vi "选择补传参数对话框.vi"() -> (3 "参数数值 2":T1)   [LabVIEW 2016, in "数据传输系统-02.lvlib"]
uses:
  <vilib>/Utility/miscctls.llb/LVPointTypeDef.ctl
panel:
  in  "取消全选":bool
  in  "取消":bool
  in  "确定":bool
  in  "全选":bool
  in  "参数数值":T2={"CODMn"=TRUE, "CODCr"=TRUE, "DO"=TRUE, "铜"=TRUE, "PH"=TRUE, "氨氮"=TRUE, "比电导率"=TRUE, "水温"=TRUE, "COD"=TRUE, "浊度"=TRUE, "总氮"=TRUE, "总磷"=TRUE, "叶绿素a"=TRUE, "藻密度"=TRUE, "水位"=TRUE, "流速"=TRUE, "瞬时流量"=TRUE, "累积流量"=TRUE, "亚硝氮"=TRUE, "硫化物"=TRUE, "ORP"=TRUE, "铅"=TRUE, "镉"=TRUE, "锌"=TRUE, "镍"=TRUE, "锰"=TRUE, "汞"=TRUE, "气温"=TRUE, "气压"=TRUE, "风速"=TRUE, "风向"=TRUE, "盐度"=TRUE, "磷酸盐"=TRUE, "硝氮"=TRUE, "氟化物"=TRUE, "挥发酚"=TRUE, "氯化物"=TRUE, "蓝绿藻"=TRUE, "余氯"=TRUE, "空气温度"=TRUE, "相对湿度"=TRUE, "分钟雨量"=TRUE, "小时雨量"=TRUE, "日雨量"=TRUE, "累积雨量"=TRUE, "方向"=TRUE, "正累积流量"=TRUE, "负累积流量"=TRUE, "综合生物毒性"=TRUE, "艏向"=TRUE, "横摇"=TRUE, "纵摇"=TRUE, "分层标志"=TRUE, "层状态1"=TRUE, "层状态2"=TRUE, "水平平均流速"=TRUE, "流向"=TRUE, "北向流速分量"=TRUE, "东向流速分量"=TRUE, "垂直流速分量"=TRUE, "最大波高"=TRUE, "最大波周期"=TRUE, "1/10波高"=TRUE, "1/10波周期"=TRUE, "有效波高"=TRUE, "有效波周期"=TRUE, "平均波高"=TRUE, "平均波周期"=TRUE, "波向"=TRUE, "波个数"=TRUE, "水深"=TRUE, "X轴流速"=TRUE, "Y轴流速"=TRUE, "信号强度"=TRUE, "电压"=TRUE, "悬浮物"=TRUE}
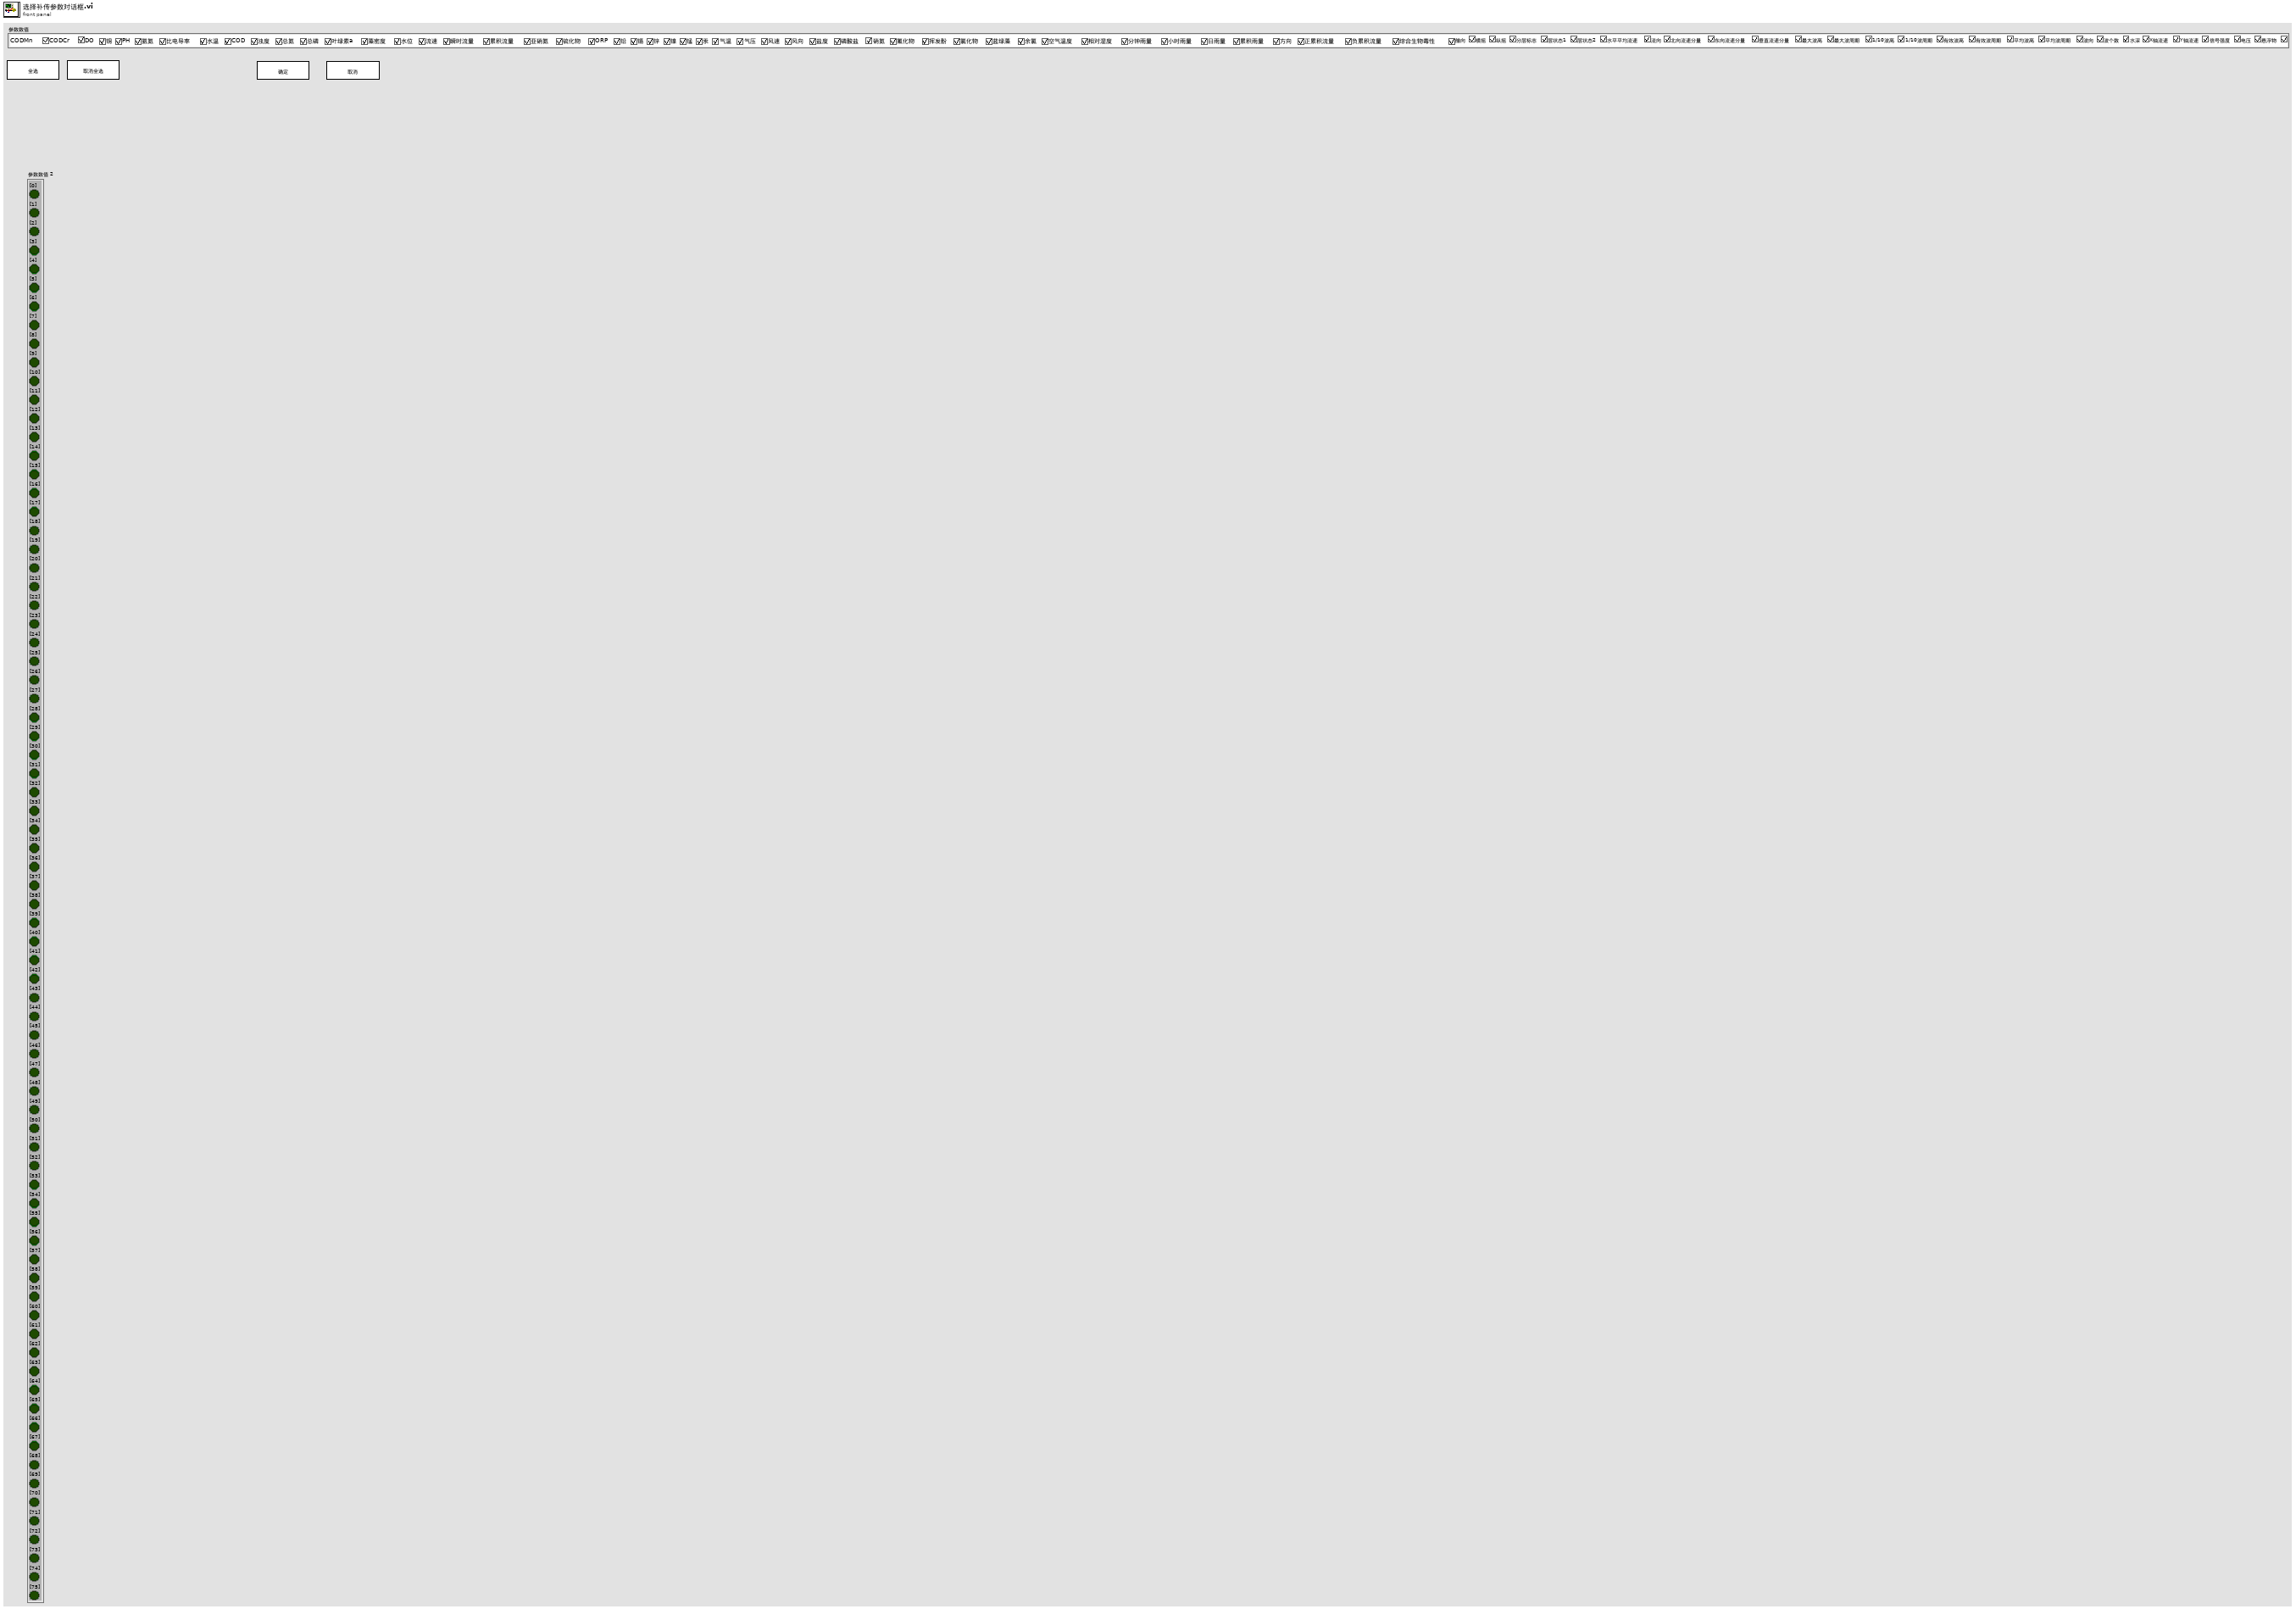
[diagram p1: front panel]
types:
  T1 = cluster{"[0]":bool, "[1]":bool, "[2]":bool, "[3]":bool, "[4]":bool, "[5]":bool, "[6]":bool, "[7]":bool, "[8]":bool, "[9]":bool, "[10]":bool, "[11]":bool, "[12]":bool, "[13]":bool, "[14]":bool, "[15]":bool, "[16]":bool, "[17]":bool, "[18]":bool, "[19]":bool, "[20]":bool, "[21]":bool, "[22]":bool, "[23]":bool, "[24]":bool, "[25]":bool, "[26]":bool, "[27]":bool, "[28]":bool, "[29]":bool, "[30]":bool, "[31]":bool, "[32]":bool, "[33]":bool, "[34]":bool, "[35]":bool, "[36]":bool, "[37]":bool, "[38]":bool, "[39]":bool, "[40]":bool, "[41]":bool, "[42]":bool, "[43]":bool, "[44]":bool, "[45]":bool, "[46]":bool, "[47]":bool, "[48]":bool, "[49]":bool, "[50]":bool, "[51]":bool, "[52]":bool, "[53]":bool, "[54]":bool, "[55]":bool, "[56]":bool, "[57]":bool, "[58]":bool, "[59]":bool, "[60]":bool, "[61]":bool, "[62]":bool, "[63]":bool, "[64]":bool, "[65]":bool, "[66]":bool, "[67]":bool, "[68]":bool, "[69]":bool, "[70]":bool, "[71]":bool, "[72]":bool, "[73]":bool, "[74]":bool, "[75]":bool}
  T2 = cluster{"CODMn":bool, "CODCr":bool, "DO":bool, "铜":bool, "PH":bool, "氨氮":bool, "比电导率":bool, "水温":bool, "COD":bool, "浊度":bool, "总氮":bool, "总磷":bool, "叶绿素a":bool, "藻密度":bool, "水位":bool, "流速":bool, "瞬时流量":bool, "累积流量":bool, "亚硝氮":bool, "硫化物":bool, "ORP":bool, "铅":bool, "镉":bool, "锌":bool, "镍":bool, "锰":bool, "汞":bool, "气温":bool, "气压":bool, "风速":bool, "风向":bool, "盐度":bool, "磷酸盐":bool, "硝氮":bool, "氟化物":bool, "挥发酚":bool, "氯化物":bool, "蓝绿藻":bool, "余氯":bool, "空气温度":bool, "相对湿度":bool, "分钟雨量":bool, "小时雨量":bool, "日雨量":bool, "累积雨量":bool, "方向":bool, "正累积流量":bool, "负累积流量":bool, "综合生物毒性":bool, "艏向":bool, "横摇":bool, "纵摇":bool, "分层标志":bool, "层状态1":bool, "层状态2":bool, "水平平均流速":bool, "流向":bool, "北向流速分量":bool, "东向流速分量":bool, "垂直流速分量":bool, "最大波高":bool, "最大波周期":bool, "1/10波高":bool, "1/10波周期":bool, "有效波高":bool, "有效波周期":bool, "平均波高":bool, "平均波周期":bool, "波向":bool, "波个数":bool, "水深":bool, "X轴流速":bool, "Y轴流速":bool, "信号强度":bool, "电压":bool, "悬浮物":bool}
  T3 = typedef "LVPointTypeDef.ctl" = cluster{"Horizontal":i16, "Vertical":i16}
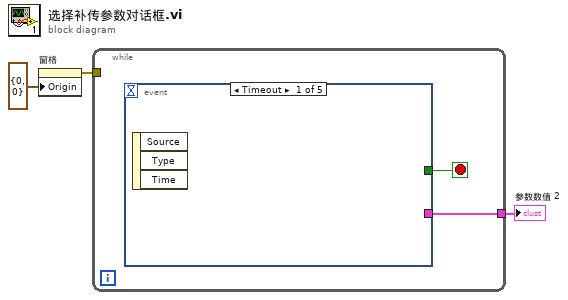
[diagram p0: block diagram]
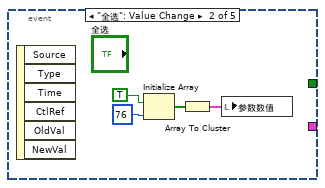
[diagram p2: hidden frame]
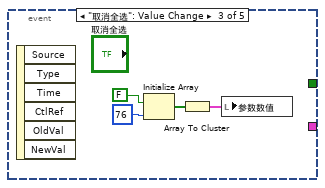
[diagram p3: hidden frame]
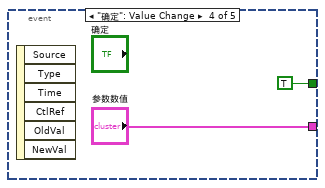
[diagram p4: hidden frame]
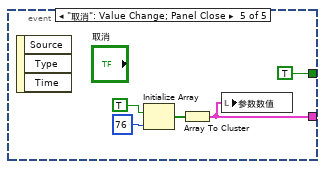
[diagram p5: hidden frame]
diagram:
  n1 = property on="窗格" class="Pane"("Origin"=T3 {"Horizontal"=0, "Vertical"=0} ("原点")) -> (error out=w2:errorcluster)  [unwired: 2 in, 1 out]
  n2 = while {
    tunnel: [w4] -> w1
    tunnel: w2 -> [_]
    stop <- w5 stop-if-true
    n3 = event shown="[0] Timeout" {
      selector: _ -> [_ _ _ _ _]
      dyn-events: _ -> [_ _ _ _ _]
      timeout: _ -> [_ _ _ _ _]
      tunnel: [_ _ _ TRUE TRUE] -> w5
      tunnel: [_ _ _ "参数数值" w16] -> w4
      event Timeout {
        n4 = event-data() -> ()  [unwired: 1 in, 3 out]
      }
      event "全选": Value Change {
        n5 = event-data() -> ()  [unwired: 1 in, 6 out]
        n6 = Initialize Array(TRUE, 76 ("维数大小")) -> (w8:bool[])
        n7 = Array To Cluster(array=w8) -> (cluster=w6:T1)
        n8 = local write "参数数值"(w6) -> ()
      }
      event "取消全选": Value Change {
        n9 = event-data() -> ()  [unwired: 1 in, 6 out]
        n10 = Initialize Array(FALSE, 76 ("维数大小")) -> (w12:bool[])
        n11 = Array To Cluster(array=w12) -> (cluster=w10:T1)
        n12 = local write "参数数值"(w10) -> ()
      }
      event "确定": Value Change {
        n13 = event-data() -> ()  [unwired: 1 in, 6 out]
      }
      event "取消": Value Change; Panel Close {
        n14 = event-data() -> ()  [unwired: 1 in, 3 out]
        n15 = Initialize Array(TRUE, 76 ("维数大小")) -> (w18:bool[])
        n16 = Array To Cluster(array=w18) -> (cluster=w16:T1)
        n17 = local write "参数数值"(w16) -> ()
      }
    }
  }
  "参数数值 2" <- w1
